vi "Delete Line.vi"(8 "error in":errorcluster, 10 "Active Line Name":string, 11 "OPC UA configuration in":refnum<class "OPC UA Server configuration.lvclass">) -> (0 "error out":errorcluster, 2 "deleted line":T1 {"OPC UA Data Type" items=["Boolean"=1, "SByte"=2, "Byte"=3, "Int16"=4, "UInt16"=5, "Int32"=6, "UInt32"=7, "Int64"=8, "UInt64"=9, "Float"=10, "Double"=11, "String"=12, "DateTime"=13, "ByteString"=15, "Array of Boolean"=101, "Array of SByte"=102, "Array of Byte"=103, "Array of Int16"=104, "Array of UInt16"=105, "Array of Int32"=106, "Array of UInt32"=107, "Array of Int64"=108, "Array of UInt64"=109, "Array of Float"=110, "Array of Double"=111, "Array of String"=112, "Array of DateTime"=113, "Array of ByteString"=115]}, 3 "OPC UA configuration out":refnum<class "OPC UA Server configuration.lvclass">)   [LabVIEW 2013, in "OPC UA Server configuration.lvclass"]
uses:
  OPC UA Server configuration.lvclass
  Line.ctl
  <vilib>/NI/Tag Bus Module Framework/channel/TBM channel.lvclass
  OPC UA Data Type.ctl
  OPC UA Server configuration.lvclass/OPC UA Server configuration.ctl
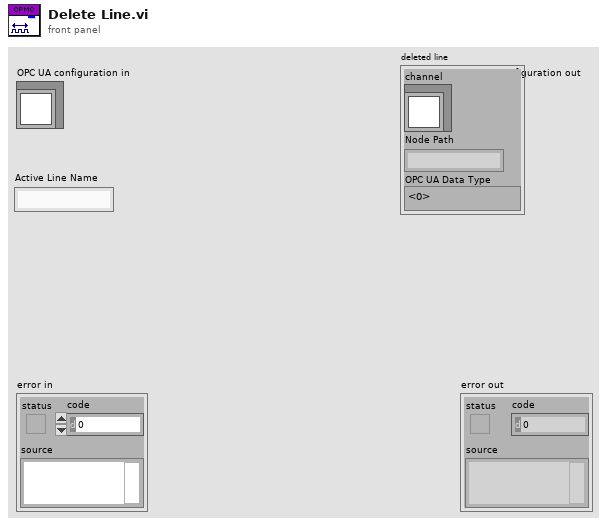
[diagram p1: front panel]
types:
  T1 = typedef "OPC UA Server configuration.lvclass/Line.ctl" = cluster{"channel":refnum<class "TBM channel.lvclass">, "Node Path":string, "OPC UA Data Type":T2}
  T2 = typedef "OPC UA Server configuration.lvclass/OPC UA Data Type.ctl" = u16
  T3 = cluster{"channel":refnum<class "TBM channel.lvclass">, "Node Path":string, "OPC UA Data Type":T2}[]
  T4 = cluster{"channel":refnum<class "TBM channel.lvclass">, "Node Path":string, "OPC UA Data Type":T2}
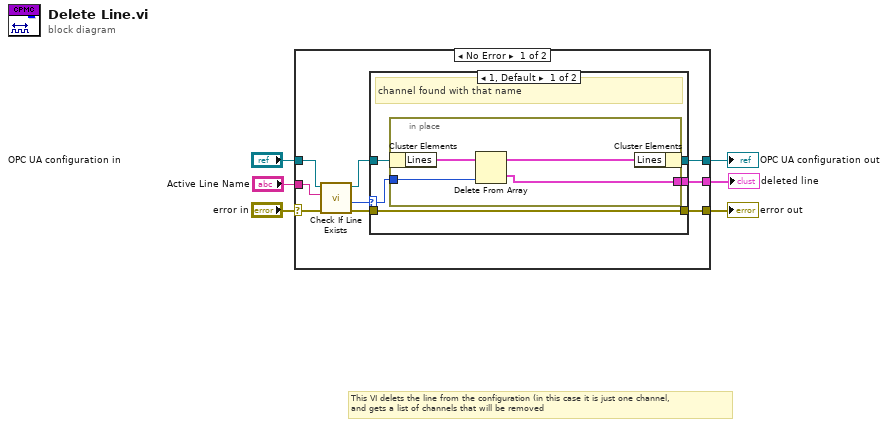
[diagram p0: block diagram]
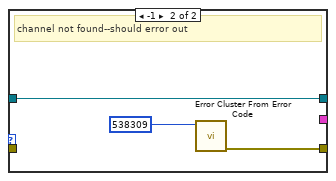
[diagram p2: hidden frame]
diagram:
  # "This VI delets the line from the configuration (in this case it is just one channel, \nand gets a list of channels that will be removed"
  n1 = case shown="No Error" "error in" {
    selector: "error in" -> [w9 w28]
    tunnel: [w15 w28] -> w6
    tunnel: [w14 w29] -> w5
    tunnel: "OPC UA configuration in" -> [w12 w29]
    tunnel: "Active Line Name" -> [w13 _]
    tunnel: [w8 _] -> w1
    frame No Error {
      n2 = call-dynamic "Check If Line Exists.vi"("error in"=w9, "name to locate"=w13, "OPC UA configuration in"=w12) -> ("error out"=w10:errorcluster, "index"=w7:i32, "OPC UA configuration out"=w11:refnum<class "OPC UA Server configuration.lvclass">)  [unwired: 4 in, 2 out]
      n3 = case shown="1, Default" w7 {
        selector: w7 -> [w16 _]
        tunnel: [w18 w27] -> w15
        tunnel: w11 -> [w20 w25]
        tunnel: [w19 w25] -> w14
        tunnel: w10 -> [w18 _]
        tunnel: [w17 _] -> w8
        frame 1, Default {
          # "channel found with that name"
          n4 = in-place {
            in-place-border: w16 -> [w24]
            in-place-border: [w21] -> w17
            n5 = in-place-cluster #1(w20) -> ("Lines"=w23:T3)
            n6 = Delete From Array(array=w23, index=w24) -> (deleted portion=w21:T4, array with subset deleted=w22:T3)  [unwired: 1 in]
            n7 = in-place-cluster #1("Lines"=w22) -> (w19:refnum<class "OPC UA Server configuration.lvclass">)
          }
        }
        frame -1 {
          # "channel not found--should error out"
          n8 = call <vilib>:"Error Cluster From Error Code.vi"("error code (0)"=538309) -> ("error out"=w27:errorcluster)  [unwired: 8 in]
        }
      }
    }
    frame Error {
    }
  }
  "error out" <- w6
  "OPC UA configuration out" <- w5
  "deleted line" <- w1
